vi "PIO.Write Byte Array.vi"(8 "error in (no error)":errorcluster, 9 "bytes to write":u8[](array[numeric]), 10 "offset":u32 format="%.0x", 11 "GE 5565PIORC in":refnum<class "GE 5565PIORC.lvclass">) -> (0 "error out":errorcluster, 3 "GE 5565PIORC out":refnum<class "GE 5565PIORC.lvclass">)   [LabVIEW 2016, in "GE 5565PIORC.lvclass"]
uses:
  GE 5565PIORC.lvclass
  GE 5565PIORC.lvclass/GE 5565PIORC.ctl
  Change Endianness (1D U32).vi
  Change Endianness (U32).vi
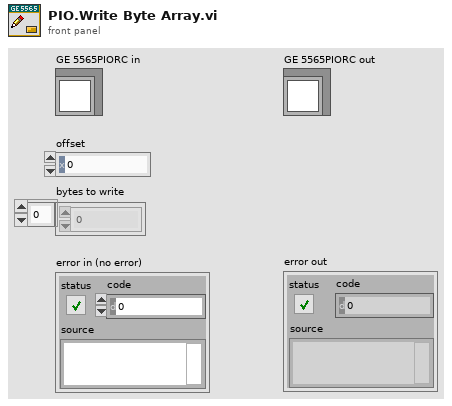
[diagram p1: front panel]
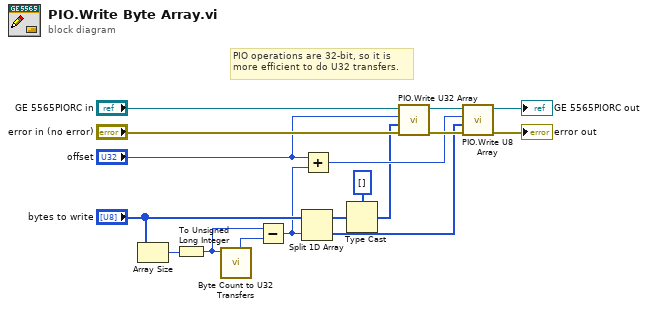
[diagram p0: block diagram]
diagram:
  # "PIO operations are 32-bit, so it is more efficient to do U32 transfers."
  n1 = Array Size(array="bytes to write") -> (size(s)=w14:i32)
  n2 = To Unsigned Long Integer(number=w14) -> (unsigned 32bit integer=w13:u32)
  n3 = call "Byte Count to U32 Transfers.vi"("bytes to transfer"=w13) -> ("U8 transfers"=w2:u32)  [unwired: 9 in, 1 out]
  n4 = Subtract(x=w13, y=w2) -> (x-y=w5:u32)
  n5 = Split 1D Array(array="bytes to write", index=w5) -> (first subarray=w7:u8[], second subarray=w3:u8[])
  n6 = Add(x="offset", y=w5) -> (x+y=w4:u32)
  n7 = Type Cast(type=u32[] [], x=w7) -> (*(type *) &x=w1:u32[])
  n8 = call "PIO.Write U32 Array.vi"("error in (no error)"="error in (no error)", "values"=w1, "offset"="offset", "GE 5565PIORC in"="GE 5565PIORC in") -> ("error out"=w10:errorcluster, "GE 5565PIORC out"=w11:refnum<class "GE 5565PIORC.lvclass">)  [unwired: 6 in]
  n9 = call "PIO.Write U8 Array.vi"("error in (no error)"=w10, "values"=w3, "offset"=w4, "GE 5565PIORC in"=w11) -> ("error out"=→"error out":errorcluster, "GE 5565PIORC out"=→"GE 5565PIORC out":refnum<class "GE 5565PIORC.lvclass">)  [unwired: 6 in]
